vi "InsertIntoSubPanel.vi"(8 "Error In":errorcluster, 10 "SubPanel in":refnum<vi>, 11 "object in":refnum<class "FrontPanelControl.lvclass">) -> (0 "Error Out":errorcluster, 3 "object out":refnum<class "FrontPanelControl.lvclass">)   [LabVIEW 2021, in "FrontPanelControl.lvclass"]
uses:
  FrontPanelControl.lvclass
  FrontPanelControl.lvclass/FrontPanelControl.ctl
  6089b93a-8969-4613-a155-0f8021851741.vi
  <vilib>/TriekselSoft/TracerLibrary/TracerLibrary/Tracer/protected/SendMessage.vi
  <vilib>/TriekselSoft/TracerLibrary/TracerLibrary/Tracer/protected/Timestamp.vi
  6089b93a-8969-4613-a155-0f8021851741.vi/f75db090-0877-4668-94fb-75c2140b1617.vi
  <vilib>/TriekselSoft/TracerLibrary/TracerLibrary/Tracer/Tracer_Level-Debug.vi
  <vilib>/JDP Science/JSONtext/Variant to JSON Text.vi
  <vilib>/TriekselSoft/TracerLibrary/TracerLibrary/Tracer/protected/Tracer_ClassAttributes.vi
  <vilib>/JDP Science/JSONtext/LVClass Serializer/JSONtext LVClass Serializer.lvclass
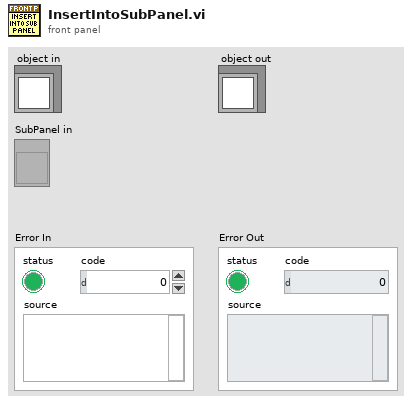
[diagram p1: front panel]
types:
  T1 = enum16{"Always On", "Always Off", "Off While Running"}
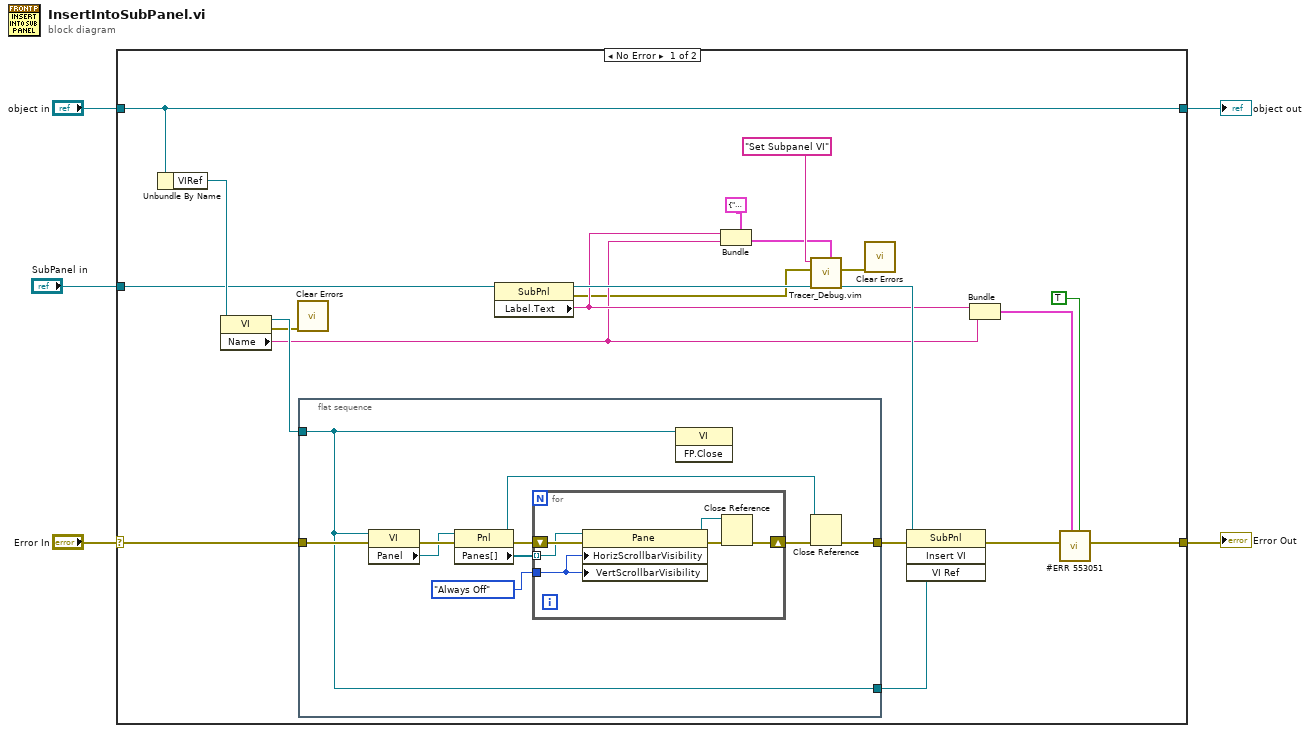
[diagram p0: block diagram]
diagram:
  n1 = case shown="No Error" "Error In" {
    selector: "Error In" -> [w22 w43]
    tunnel: [w18 w43] -> w4
    tunnel: [w25 w42] -> w2
    tunnel: "object in" -> [w25 w42]
    tunnel: "SubPanel in" -> [w20 _]
    frame No Error {
      n2 = Unbundle By Name(w25) -> ("VIRef"=w23:refnum<vi>)
      n3 = property class="VI"(reference=w23) -> (reference out=w15:refnum<vi>, error out=w13:errorcluster, "Name"=w10:string)  [unwired: 1 in]
      n4 = call <vilib>:"Clear Errors.vi"("error in (no error)"=w13) -> ()  [unwired: 5 in, 2 out]
      n5 = flat-sequence {
        tunnel: w15 -> [w26]
        tunnel: [w26] -> w24
        tunnel: [w28] -> w21
        tunnel: w22 -> [w35]
        frame #0 {
          n6 = property class="VI"(reference=w26, error in=w35) -> (error out=w34:errorcluster, "Panel"=w33:refnum<vi>)  [unwired: 1 out]
          n7 = property class="Pnl"(reference=w33, error in=w34) -> (reference out=w27:refnum<vi>, error out=w32:errorcluster, "Panes[]"=w31:refnum<vi>[])
          n8 = for {
            shift-right: [w37] -> w29
            shift-left: w32 -> [w41]
            tunnel: w31 -> [w39] mode=indexing
            tunnel: T1."Always Off" ("Vertical Scrollbar Visibility") -> [w38]
            n9 = property class="Pane"(reference=w39, error in=w41, "HorizScrollbarVisibility"=w38, "VertScrollbarVisibility"=w38) -> (reference out=w36:refnum<vi>, error out=w40:errorcluster)
            n10 = Close Reference(reference=w36, error in (no error)=w40) -> (error out=w37:errorcluster)
          }
          n11 = invoke class="VI" method="FP.Close"(reference=w26) -> ()  [unwired: 2 in, 3 out]
          n12 = Close Reference(reference=w27, error in (no error)=w29) -> (error out=w28:errorcluster)
        }
      }
      n13 = property class="SubPnl"(reference=w20) -> (reference out=w16:refnum<vi>, error out=w8:errorcluster, "Label.Text"=w11:string)  [unwired: 1 in]
      n14 = Bundle(cluster=cluster{"SubPanelLabel":string, "VIName":string} {"SubPanelLabel"="", "VIName"=""}, "SubPanelLabel"=w11, "VIName"=w10) -> (w9:cluster{"SubPanelLabel":string, "VIName":string})
      n15 = call "Tracer_Debug.vim"("Data"=w9, "error in (no error)"=w8, "Text"="Set Subpanel VI") -> ("error out"=w7:errorcluster)  [unwired: 8 in]
      n16 = call <vilib>:"Clear Errors.vi"("error in (no error)"=w7) -> ()  [unwired: 5 in, 2 out]
      n17 = invoke class="SubPnl" method="Insert VI"(reference=w16, error in=w21, "VI Ref"=w24) -> (error out=w19:errorcluster)  [unwired: 1 in, 3 out]
      n18 = Bundle("Label.Text"=w11, "Name"=w10) -> (w14:cluster{"Label.Text":string, "Name":string})  [unwired: 1 in]
      n19 = call "#ERR 553051"("MergeErrors"=TRUE, "Data"=w14, "error in (no error)"=w19) -> ("error out"=w18:errorcluster)  [unwired: 8 in]
    }
    frame Error {
    }
  }
  "Error Out" <- w4
  "object out" <- w2
